vi "Keysight_N6700C_Measure.vi"(8 "error in (no error)":errorcluster, 10 "Channel Name (1)":string="1", 11 "VISA resource name":refnum<visa-resource-name>) -> (0 "error out":errorcluster, 1 "Current":dbl format="%^.3e", 2 "Voltage":dbl format="%^.3e", 3 "VISA resource name out":refnum<visa-resource-name>)   [LabVIEW 2018]
uses:
  SupportVIs/Agilent N6700 Series.lvlib
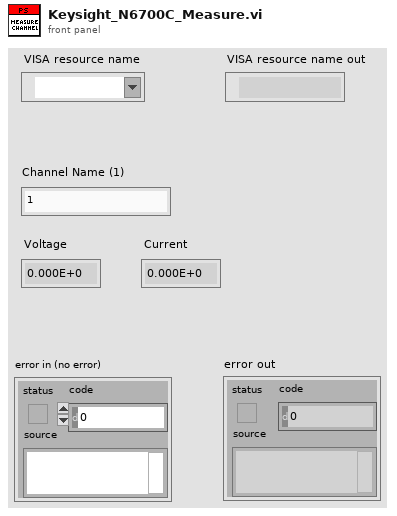
[diagram p1: front panel]
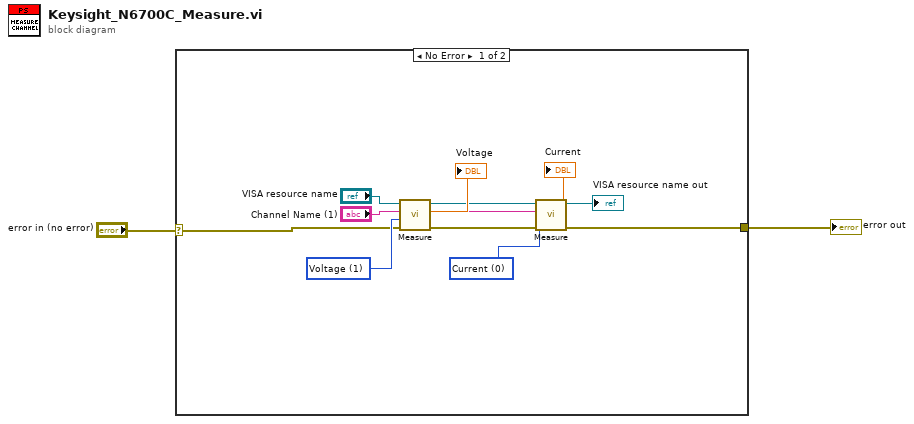
[diagram p0: block diagram]
diagram:
  n1 = case shown="No Error" "error in (no error)" {
    selector: "error in (no error)" -> [w11 w14]
    tunnel: [w3 w14] -> w2
    frame No Error {
      w8 = 0 items=["Current", "Voltage", "Power"] ("Measurement Type (1: Voltage)")
      w12 = 1 items=["Current", "Voltage", "Power"] ("Measurement Type (1: Voltage)")
      n2 = call "Measure.vi"("error in (no error)"=w11, "Measurement Type (1: Voltage)"=w12, "Channel Name (1)"="Channel Name (1)", "VISA resource name"="VISA resource name") -> ("error out"=w7:errorcluster, "Measurement"=→"Voltage":dbl, "VISA resource name out"=w9:refnum<visa-resource-name>)  [unwired: 5 in]
      n3 = call "Measure.vi"("error in (no error)"=w7, "Measurement Type (1: Voltage)"=w8, "Channel Name (1)"="Channel Name (1)", "VISA resource name"=w9) -> ("error out"=w3:errorcluster, "Measurement"=→"Current":dbl, "VISA resource name out"=→"VISA resource name out":refnum<visa-resource-name>)  [unwired: 5 in]
    }
    frame Error {
    }
  }
  "error out" <- w2
